vi "zmq_z85_decode.vi"(3 "error in":errorcluster, 5 "encoded string":string) -> (0 "error out":errorcluster, 2 "data out":u8[](array[numeric]))   [LabVIEW 2019, in "zeromq.lvlib"]
doc: "Queries and returns the version of ZeroMQ currently loaded as both a string and struct.\n\nDetailed API documentation: http://api.zeromq.org/3-2:zmq-version"
uses:
  zeromq.lvlib
panel:
  # "ØMQ"
  # "labview"
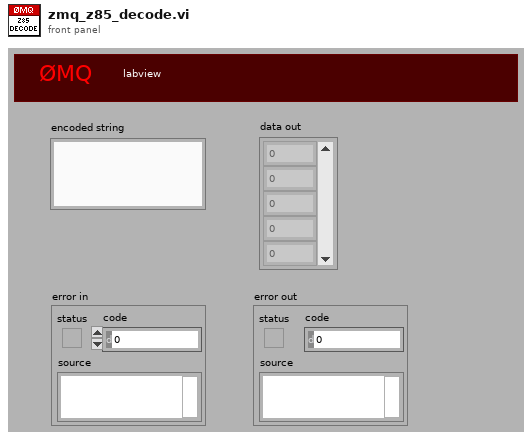
[diagram p1: front panel]
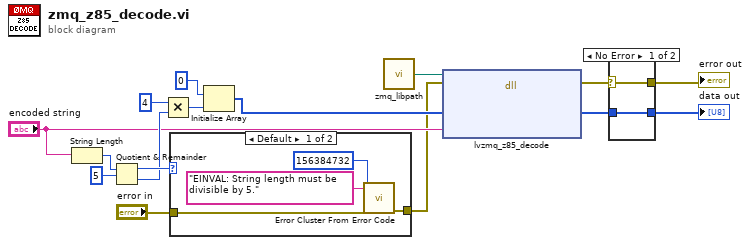
[diagram p0: block diagram]
diagram:
  n1 = String Length(string="encoded string") -> (length=w7:i32)
  n2 = Quotient & Remainder(x=w7, y=5) -> (x-y*floor(x/y)=w12:i32, floor(x/y)=w11:i32)
  n3 = Multiply(x=4, y=w11) -> (x*y=w9:i32)
  n4 = case shown="Default" w12 {
    tunnel: "error in" -> [w18 w21]
    tunnel: [w17 w21] -> w5
    frame Default {
      n5 = call <vilib>:"Error Cluster From Error Code.vi"("error in (no error)"=w18, "error message (\"\")"="EINVAL: String length must be divisible by 5." ("error message (\"\")"), "error code (0)"=156384732) -> ("error out"=w17:errorcluster)  [unwired: 6 in]
    }
    frame 0 {
      # "Divisible by 5, is ok"
    }
  }
  n6 = Initialize Array(u8 0 ("element"), w9) -> (w13:u8[])
  n7 = call "zmq_libpath.vi"() -> ("path"=w16:path)
  n8 = dll-call lib="?" fn="lvzmq_z85_decode" ("zmq_labview.dll:lvzmq_socket")(path in=w16, error in=w5, "dest"=w13, "src"="encoded string") -> (error out=w4:errorcluster, "dest"=w2:u8[])  [unwired: 3 in, 1 out]
  n9 = case shown="No Error" w4 {
    selector: w4 -> [w23 w24]
    tunnel: [w23 w24] -> w3
    tunnel: [w22 _] -> w1
    tunnel: w2 -> [w22 _]
    frame No Error {
    }
    frame Error {
    }
  }
  "error out" <- w3
  "data out" <- w1
